vi "running.get.vi"(11 "manager_daemon in":refnum<class "manager_daemon.lvclass">) -> (2 "manager running":bool, 3 "manager daemon":refnum<class "manager_daemon.lvclass">)   [LabVIEW 2024, in "manager_daemon.lvclass"]
uses:
  manager_daemon.lvclass
  manager_daemon.lvclass/manager_daemon.ctl
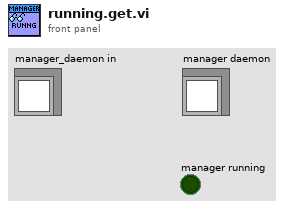
[diagram p1: front panel]
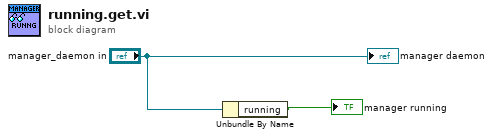
[diagram p0: block diagram]
diagram:
  n1 = Unbundle By Name("manager_daemon in") -> ("running"=→"manager running":bool)
  "manager daemon" <- "manager_daemon in"
